vi "Command Byte.vi"(10 "Command":T1) -> (2 "Command Byte":string)   [LabVIEW 2020, in "FormulaG.lvlib" / "FormulaG API.lvclass"]
uses:
  FormulaG API.lvclass
  Command.ctl
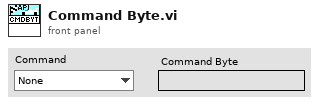
[diagram p1: front panel]
types:
  T1 = typedef "FormulaG.lvlib/FormulaG API.lvclass/Command.ctl" = enum8{"None", "Reset Car", "Request State", "Control Car", "Request Info", "Set Options", "Set Camera", "Set Pause", "Request Time"}
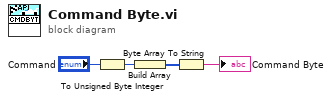
[diagram p0: block diagram]
diagram:
  n1 = To Unsigned Byte Integer(number="Command") -> (unsigned 8bit integer=w3:u8)
  n2 = Build Array(w3) -> (w2:u8[])
  n3 = Byte Array To String(unsigned byte array=w2) -> (string=→"Command Byte":string)
